vi "PL Model.vi"(7 "PL Model Exit":refnum<notifier>, 8 "error in (no error)":errorcluster, 10 "Controller queue":refnum<queue>, 11 "Message Queue In":refnum<queue>) -> (0 "error out":errorcluster)   [LabVIEW 2015, in "PL Model.lvlib"]
uses:
  PL Model.lvlib
  support/Message Queue/Message Cluster.ctl
  TypeDefs/UI/Line simulation.ctl
  TypeDefs/PL Model Data.ctl
  TypeDefs/PL Settings.ctl
  TypeDefs/PL UI Refs.ctl
  API/Get Model Status Control.ctl
  SubVIs/Global Data.vi
  support/Message Queue/Enqueue Message (Single).vi
  <vilib>/Utility/error.llb/Error Cluster From Error Code.vi
  <vilib>/ErrorRing/Error Ring.xnode
  support/Message Queue/PLC Message Queue.lvlib
  support/Message Queue/Message Queue.lvlib
panel:
  out "PL Model counter":i32
  out "Barrel Number":i32
  out "BARREL FILLED":bool
  out "SPILL ALARM":bool
  out "OUTPUT":bool
  out "DOSING":bool
  out "INPUT":bool
  out "Flow [l/s]":dbl(knob) scale=0.0..30.0
  out "Fluid Level [l]":dbl(slide) scale=0.0..100.0
  out "Production line":T1 max=100.0 scale=0.0..20.0
  out "Pump":bool
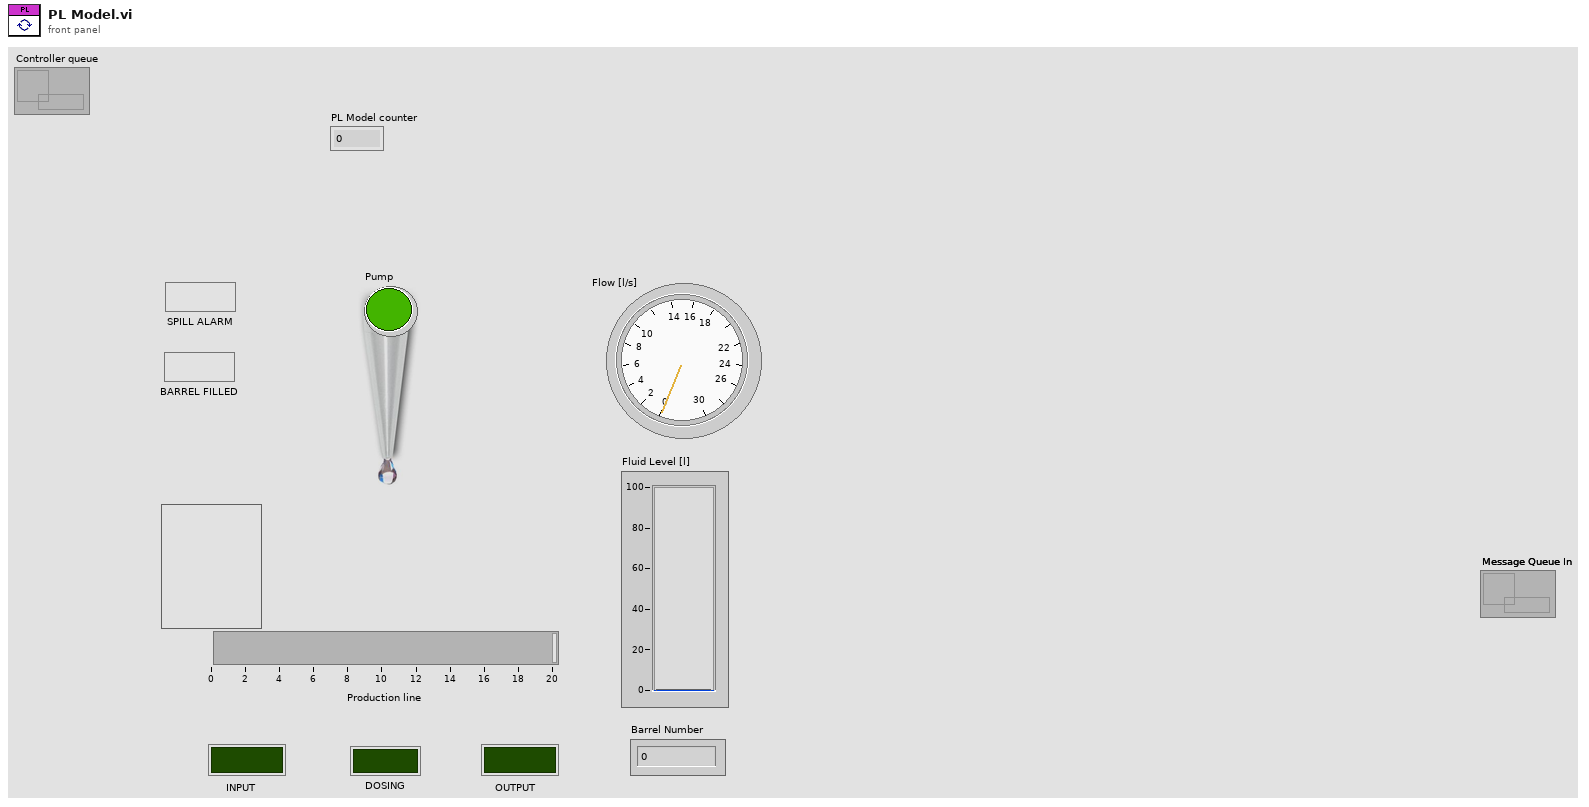
[diagram p1: front panel]
types:
  T1 = typedef "PL Model.lvlib/Line simulation.ctl" = dbl
  T2 = typedef "PL Model.lvlib/PL Model Data.ctl" = cluster{"Position":dbl, "Settings":T3, "Pump State":bool, "Fluid Flow":dbl, "Inpute Zone":bool, "Dosing Zone":bool, "Output Zone":bool, "UI Refs":T4, "Fluid Level":dbl, "Barrel Number":i32, "Spill Alarm":bool, "Level Alarm":bool, "millisecond timer value":u32}
  T3 = typedef "PL Model.lvlib/PL Settings.ctl" = cluster{"Length [m]":dbl, "Dose Zone Start":dbl, "Dose Zone  End":dbl, "Barrel Volume [l]":dbl, "Dosing level [l]":dbl}
  T4 = typedef "PL Model.lvlib/PL UI Refs.ctl" = cluster{"DOSING":refnum<vi>, "INPUT":refnum<vi>, "OUTPUT":refnum<vi>, "Pump":refnum<vi>, "Fluid Level [l]":refnum<vi>, "Flow [l/s]":refnum<vi>, "Production line":refnum<vi>, "SPILL":refnum<vi>, "LOW LEVEL":refnum<vi>, "Barrel Number":refnum<vi>}
  T5 = typedef "PL Model.lvlib/Get Model Status Control.ctl" = cluster{"Position":dbl, "Pump State":bool, "Fluid Flow":dbl, "Fluid Level":dbl, "Barrel Number":i32, "Spill Alarm":bool, "Level Alarm":bool}
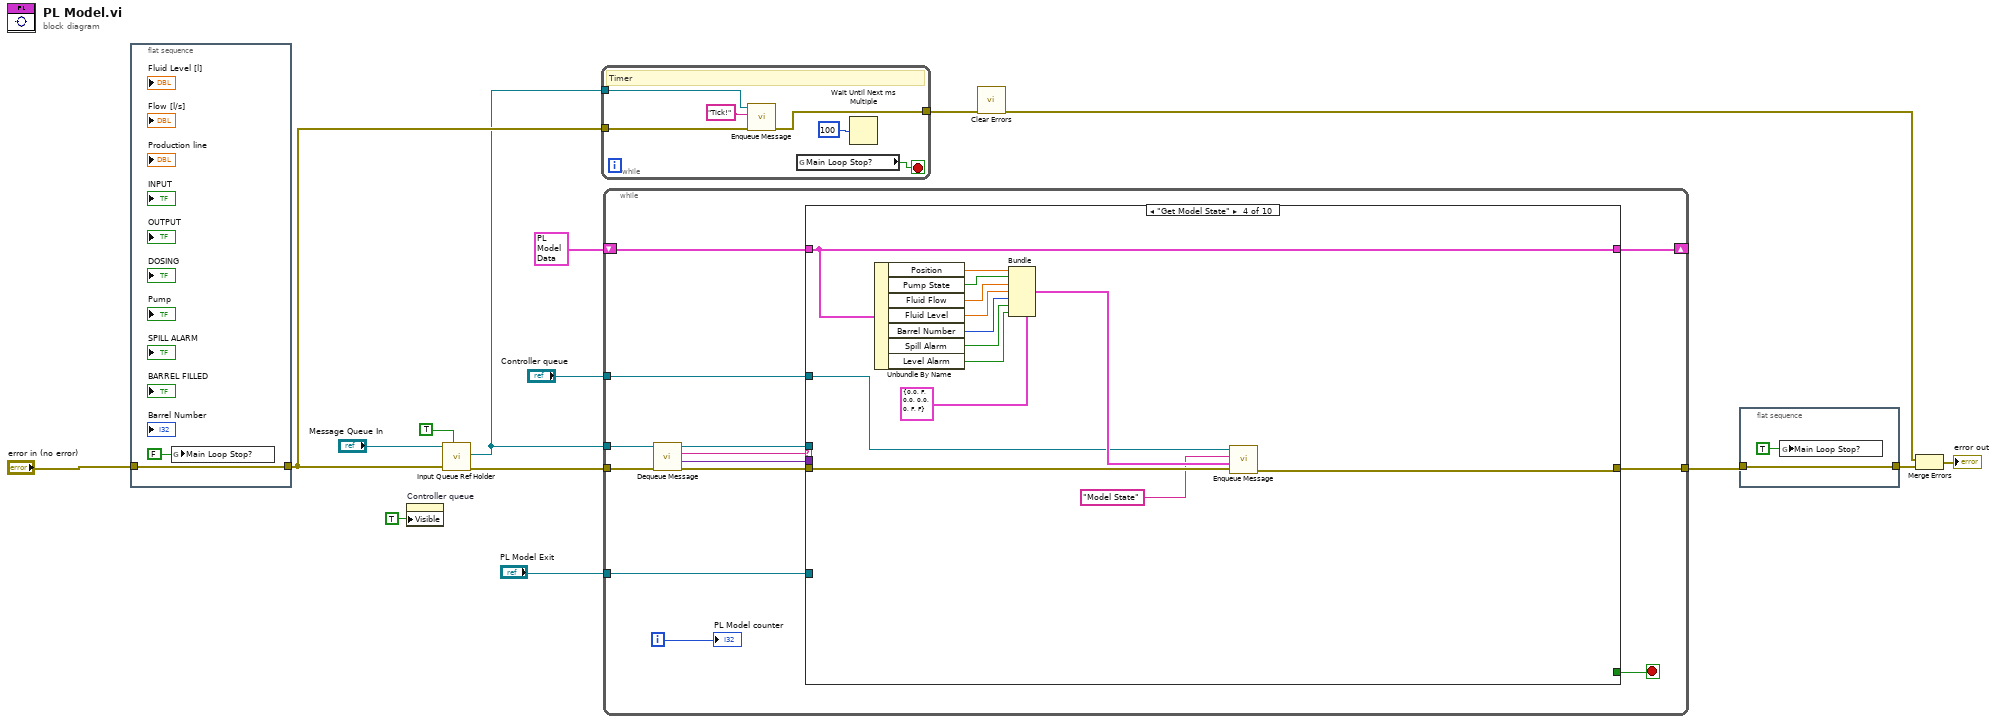
[diagram p0: block diagram]
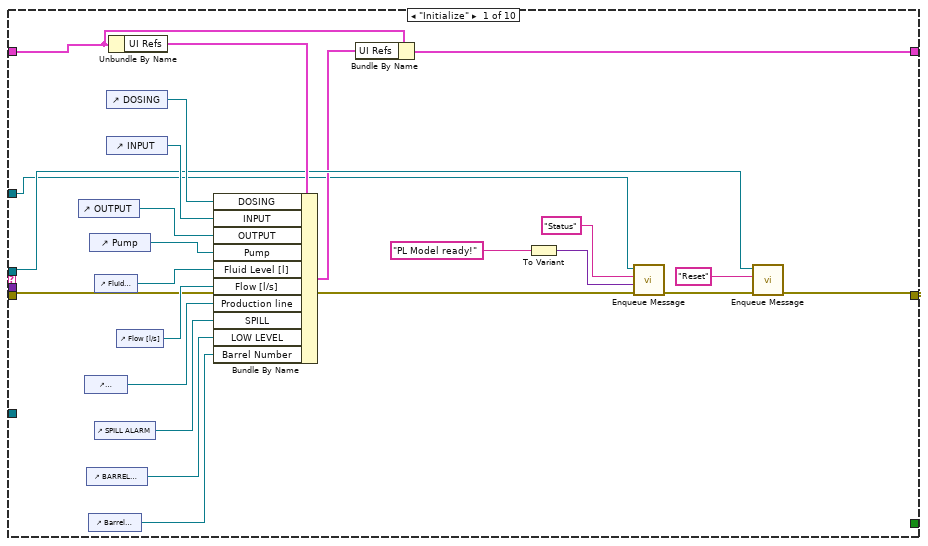
[diagram p2: hidden frame]
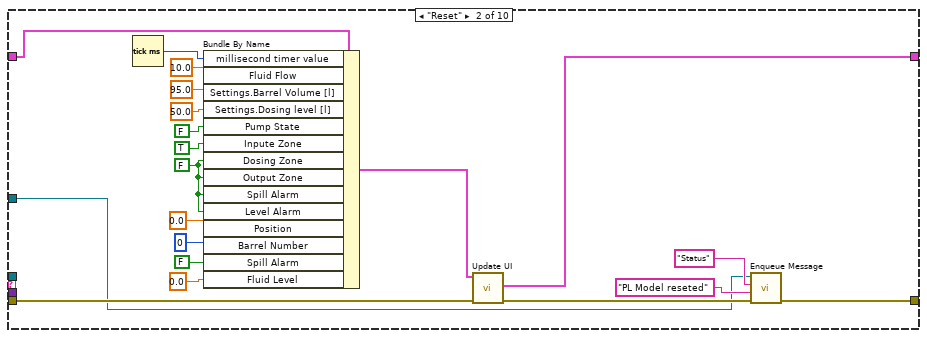
[diagram p3: hidden frame]
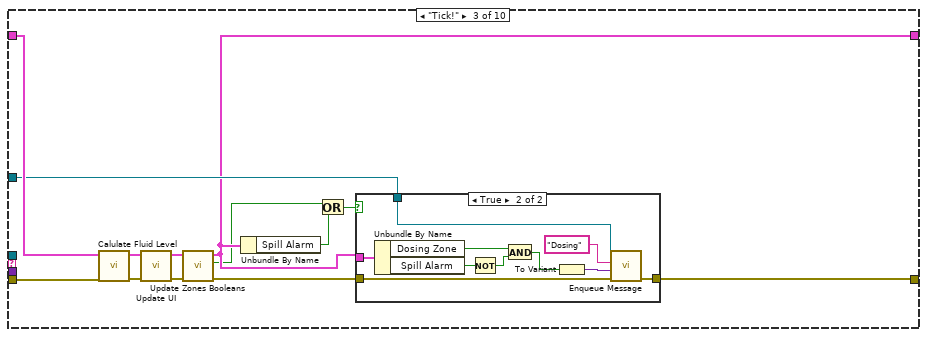
[diagram p4: hidden frame]
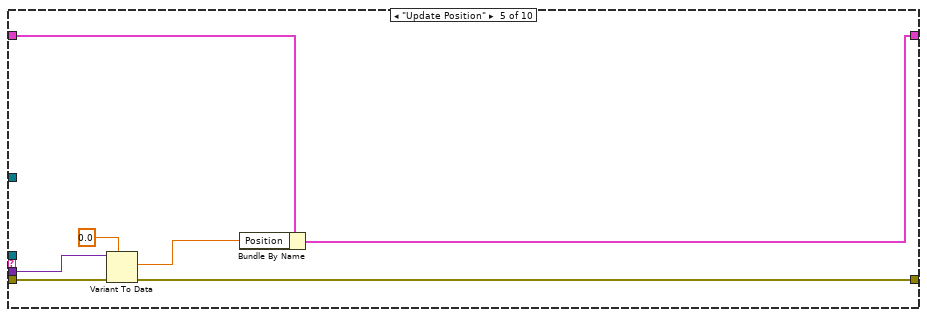
[diagram p6: hidden frame]
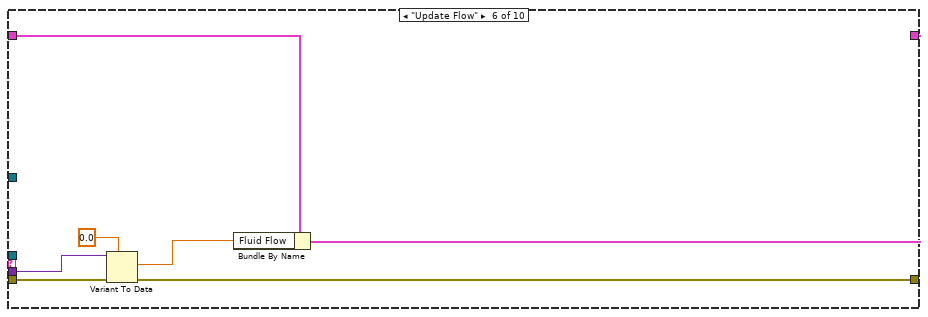
[diagram p7: hidden frame]
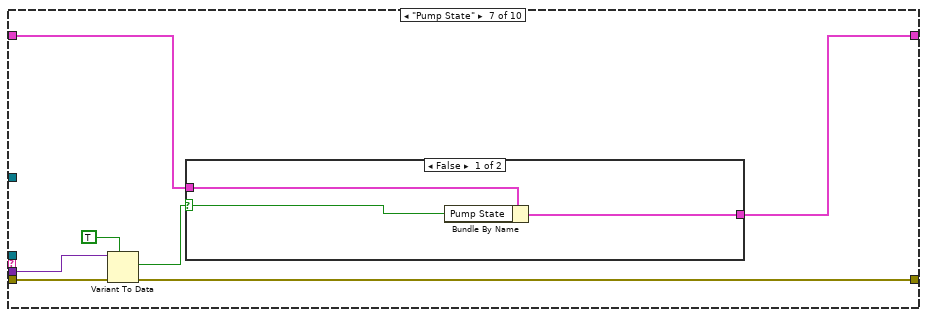
[diagram p8: hidden frame]
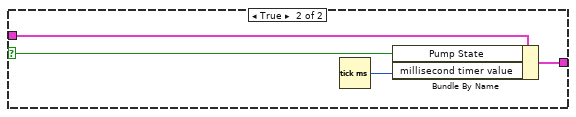
[diagram p9: hidden frame]
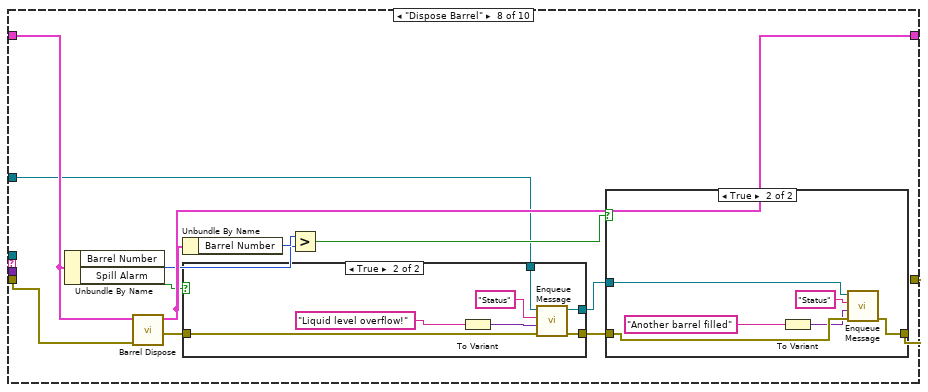
[diagram p10: hidden frame]
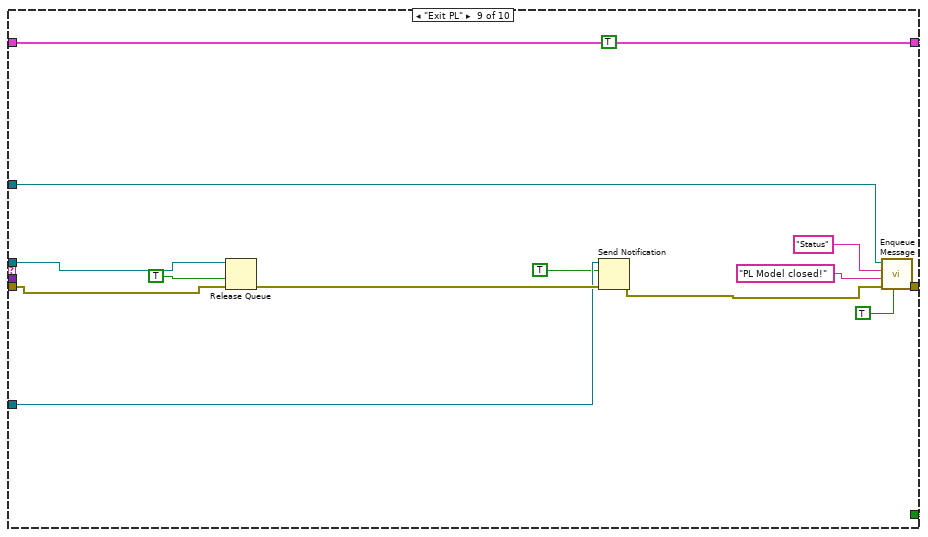
[diagram p13: hidden frame]
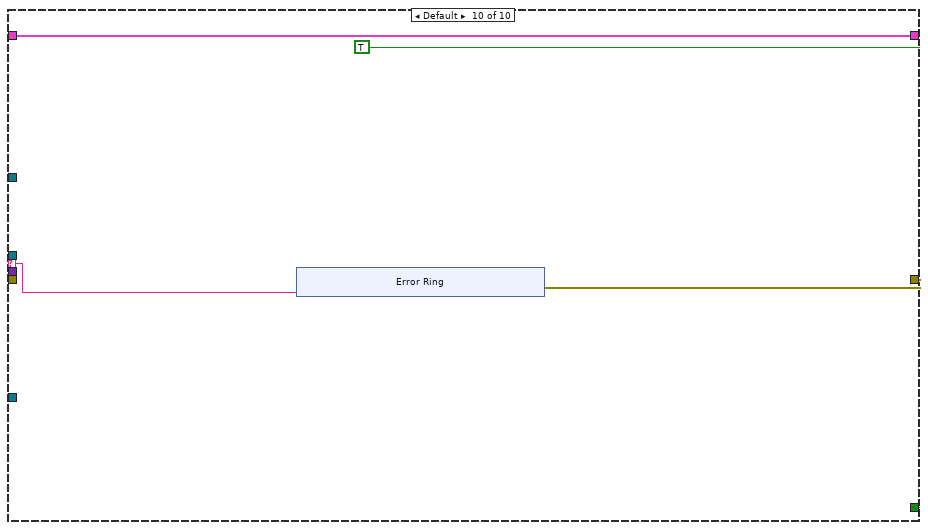
[diagram p14: hidden frame]
diagram:
  n1 = flat-sequence {
    tunnel: "error in (no error)" -> [w16]
    tunnel: [w16] -> w10
    frame #0 {
      n2 = global write "Global Data.vi" "Main Loop Stop?"(FALSE ("Main Loop Stop?")) -> ()
    }
  }
  n3 = property on="Controller queue" class="TypRef (strict)"("Visible"=TRUE) -> ()  [unwired: 2 in, 2 out]
  n4 = call "Input Queue Ref Holder.vi"("Hold"=TRUE, "error in (no error)"=w10, "Message Queue In"="Message Queue In") -> ("error out"=w9:errorcluster, "Input Message Queue"=w6:refnum<queue>)  [unwired: 7 in]
  n5 = while {
    tunnel: w6 -> [w21]
    tunnel: [w20] -> w3
    tunnel: w10 -> [w18]
    stop <- w22 stop-if-true
    # "Timer"
    n6 = call-poly "Enqueue Message.vi"("error in (no error)"=w18, "Message"="Tick!", "Message Queue"=w21) -> ("error out"=w20:errorcluster)  [unwired: 7 in, 1 out]
    n7 = global read "Global Data.vi" "Main Loop Stop?"() -> (w22:bool)
    n8 = Wait Until Next ms Multiple(millisecond multiple=u32 100) -> ()  [unwired: 1 out]
  }
  n9 = while {
    tunnel: w6 -> [w36]
    shift-right: [w28] -> _
    shift-left: T2 {"Position"=0.0, "Settings"={"Length [m]"=20.0, "Dose Zone Start"=8.0, "Dose Zone  End"=12.0, "Barrel Volume [l]"=100.0, "Dosing level [l]"=90.0}, "Pump State"=FALSE, "Fluid Flow"=0.0, "Inpute Zone"=FALSE, "Dosing Zone"=FALSE, "Output Zone"=FALSE, "UI Refs"={"DOSING"=refnum, "INPUT"=refnum, "OUTPUT"=refnum, "Pump"=refnum, "Fluid Level [l]"=refnum, "Flow [l/s]"=refnum, "Production line"=refnum, "SPILL"=refnum, "LOW LEVEL"=refnum, "Barrel Number"=refnum}, "Fluid Level"=0.0, "Barrel Number"=0, "Spill Alarm"=FALSE, "Level Alarm"=FALSE, "millisecond timer value"=0} ("PL Model Data") -> [w29]
    tunnel: [w34] -> w13
    tunnel: w9 -> [w33]
    tunnel: "PL Model Exit" -> [w26]
    tunnel: "Controller queue" -> [w25]
    i -> [w24]
    stop <- w27 stop-if-true
    n10 = call "Dequeue Message.vi"("error in (no error)"=w33, "Message Queue"=w36) -> ("error out"=w35:errorcluster, "Message Data"=w31:variant, "Message"=w32:string, "dup Message Queue"=w30:refnum<queue>)  [unwired: 6 in]
    n11 = case shown="\"Get Model State\"" w32 {
      selector: w32 -> [_ _ _ _ _ _ _ _ _ w191]
      tunnel: w35 -> [w37 w67 w92 w109 w124 w131 w138 w157 w185 _]
      tunnel: [w42 w68 w85 w108 w118 w125 w133 w156 w177 w190] -> w34
      tunnel: w31 -> [_ _ _ _ w123 w130 w137 _ _ _]
      tunnel: w30 -> [w44 _ _ _ _ _ _ _ w184 _]
      tunnel: w29 -> [w40 w79 w91 w107 w122 w129 w136 w155 w187 w188]
      tunnel: [w39 w65 w84 w107 w121 w128 w135 w154 w187 w188] -> w28
      tunnel: [_ _ _ _ _ _ _ _ TRUE TRUE] -> w27
      tunnel: w26 -> [_ _ _ _ _ _ _ _ w182 _]
      tunnel: w25 -> [w38 w60 w87 w105 _ _ _ w146 w174 _]
      frame "Initialize" {
        n12 = control-ref of="OUTPUT"() -> (w55:refnum<vi>)
        n13 = control-ref of="Production line"() -> (w59:refnum<vi>)
        n14 = control-ref of="BARREL FILLED"() -> (w51:refnum<vi>)
        n15 = control-ref of="Barrel Number"() -> (w49:refnum<vi>)
        n16 = control-ref of="Pump"() -> (w56:refnum<vi>)
        n17 = control-ref of="Fluid Level [l]"() -> (w57:refnum<vi>)
        n18 = control-ref of="SPILL ALARM"() -> (w50:refnum<vi>)
        n19 = control-ref of="DOSING"() -> (w53:refnum<vi>)
        n20 = control-ref of="INPUT"() -> (w54:refnum<vi>)
        n21 = Unbundle By Name(w40) -> ("UI Refs"=w52:T4)
        n22 = control-ref of="Flow [l/s]"() -> (w58:refnum<vi>)
        n23 = Bundle By Name(cluster=w52, "DOSING"=w53, "INPUT"=w54, "OUTPUT"=w55, "Pump"=w56, "Fluid Level [l]"=w57, "Flow [l/s]"=w58, "Production line"=w59, "SPILL"=w50, "LOW LEVEL"=w51, "Barrel Number"=w49) -> (w41:T4)
        n24 = Bundle By Name(cluster=w40, "UI Refs"=w41) -> (w39:T2)
        n25 = To Variant(anything="PL Model ready!" ("Message")) -> (Variant=w46:variant)
        n26 = call-poly "Enqueue Message.vi"("error in (no error)"=w37, "Message Data"=w46, "Message"="Status", "Message Queue"=w38) -> ("error out"=w45:errorcluster)  [unwired: 6 in, 1 out]
        n27 = call-poly "Enqueue Message.vi"("error in (no error)"=w45, "Message"="Reset", "Message Queue"=w44) -> ("error out"=w42:errorcluster)  [unwired: 7 in, 1 out]
      }
      frame "Reset" {
        w71 = FALSE ("Inpute Zone")
        n28 = Tick Count (ms)() -> (millisecond timer value=w76:u32)
        n29 = Bundle By Name(cluster=w79, "millisecond timer value"=w76, "Fluid Flow"=10.0, "Settings.Barrel Volume [l]"=95.0, "Settings.Dosing level [l]"=50.0, "Pump State"=FALSE, "Inpute Zone"=TRUE, "Dosing Zone"=w71, "Output Zone"=w71, "Spill Alarm"=w71, "Level Alarm"=w71, "Position"=0.0, "Barrel Number"=0, "Spill Alarm"=FALSE, "Fluid Level"=0.0) -> (w69:T2)
        n30 = call "Update UI.vi"("error in (no error)"=w67, "PL Model Data"=w69) -> ("error out"=w66:errorcluster, "PL Model Data"=w65:T2)  [unwired: 8 in]
        n31 = call-poly "Enqueue Message.vi"("error in (no error)"=w66, "Message Data"="PL Model reseted" ("Message"), "Message"="Status", "Message Queue"=w60) -> ("error out"=w68:errorcluster)  [unwired: 6 in, 1 out]
      }
      frame "Tick!" {
        n32 = call "Calulate Fluid Level.vi"("error in (no error)"=w92, "PL Model Data"=w91) -> ("error out"=w90:errorcluster, "PL Model Data Out"=w80:T2)  [unwired: 8 in]
        n33 = call "Update UI.vi"("error in (no error)"=w90, "PL Model Data"=w80) -> ("error out"=w89:errorcluster, "PL Model Data"=w88:T2)  [unwired: 8 in]
        n34 = call "Update Zones Booleans.vi"("error in (no error)"=w89, "PL Model Data"=w88) -> ("error out"=w86:errorcluster, "Zone change?"=w83:bool, "PL Model Data 2"=w84:T2)  [unwired: 7 in]
        n35 = Unbundle By Name(w84) -> ("Spill Alarm"=w81:bool)
        n36 = Or(x=w83, y=w81) -> (x .or. y?=w82:bool)
        n37 = case shown="True" w82 {
          tunnel: w84 -> [_ w103]
          tunnel: w87 -> [_ w102]
          tunnel: w86 -> [w93 w101]
          tunnel: [w93 w94] -> w85
          frame False {
          }
          frame True {
            n38 = Unbundle By Name(w103) -> ("Dosing Zone"=w96:bool, "Spill Alarm"=w98:bool)
            n39 = Not(x=w98) -> (.not. x?=w97:bool)
            n40 = And(x=w96, y=w97) -> (x .and. y?=w95:bool)
            n41 = To Variant(anything=w95) -> (Variant=w100:variant)
            n42 = call-poly "Enqueue Message.vi"("error in (no error)"=w101, "Message Data"=w100, "Message"="Dosing", "Message Queue"=w102) -> ("error out"=w94:errorcluster)  [unwired: 6 in, 1 out]
          }
        }
      }
      frame "Get Model State" {
        n43 = Unbundle By Name(w107) -> ("Position"=w117:dbl, "Pump State"=w116:bool, "Fluid Flow"=w115:dbl, "Fluid Level"=w114:dbl, "Barrel Number"=w113:i32, "Spill Alarm"=w112:bool, "Level Alarm"=w111:bool)
        n44 = Bundle(cluster=T5 {"Position"=0.0, "Pump State"=FALSE, "Fluid Flow"=0.0, "Fluid Level"=0.0, "Barrel Number"=0, "Spill Alarm"=FALSE, "Level Alarm"=FALSE} ("output cluster"), "Position"=w117, "Pump State"=w116, "Fluid Flow"=w115, "Fluid Level"=w114, "Barrel Number"=w113, "Spill Alarm"=w112, "Level Alarm"=w111) -> (w106:T5)
        n45 = call-poly "Enqueue Message.vi"("error in (no error)"=w109, "Message Data"=w106, "Message"="Model State", "Message Queue"=w105) -> ("error out"=w108:errorcluster)  [unwired: 6 in, 1 out]
      }
      frame "Update Position" {
        n46 = Variant To Data(error in=w124, type=0.0, Variant=w123) -> (data=w119:dbl, error out=w118:errorcluster)
        n47 = Bundle By Name(cluster=w122, "Position"=w119) -> (w121:T2)
      }
      frame "Update Flow" {
        n48 = Variant To Data(error in=w131, type=0.0, Variant=w130) -> (data=w126:dbl, error out=w125:errorcluster)
        n49 = Bundle By Name(cluster=w129, "Fluid Flow"=w126) -> (w128:T2)
      }
      frame "Pump State" {
        n50 = Variant To Data(error in=w138, type=TRUE, Variant=w137) -> (data=w132:bool, error out=w133:errorcluster)
        n51 = case shown="False" w132 {
          selector: w132 -> [w139 w142]
          tunnel: w136 -> [w141 w145]
          tunnel: [w140 w144] -> w135
          frame False {
            n52 = Bundle By Name(cluster=w141, "Pump State"=w139) -> (w140:T2)
          }
          frame True {
            n53 = Tick Count (ms)() -> (millisecond timer value=w143:u32)
            n54 = Bundle By Name(cluster=w145, "Pump State"=w142, "millisecond timer value"=w143) -> (w144:T2)
          }
        }
      }
      frame "Dispose Barrel" {
        n55 = Unbundle By Name(w155) -> ("Barrel Number"=w152:i32, "Spill Alarm"=w147:bool)
        n56 = call "Barrel Dispose.vi"("error in (no error)"=w157, "PL Model Data in"=w155) -> ("error out"=w149:errorcluster, "PL Model Data out"=w154:T2)  [unwired: 8 in]
        n57 = Unbundle By Name(w154) -> ("Barrel Number"=w153:i32)
        n58 = case shown="True" w147 {
          tunnel: w149 -> [w159 w164]
          tunnel: [w159 w163] -> w148
          tunnel: [w158 w162] -> w150
          tunnel: w146 -> [w158 w160]
          frame False {
          }
          frame True {
            n59 = To Variant(anything="Liquid level overflow!" ("Message")) -> (Variant=w161:variant)
            n60 = call-poly "Enqueue Message.vi"("error in (no error)"=w164, "Message Data"=w161, "Message"="Status", "Message Queue"=w160) -> ("error out"=w163:errorcluster, "dup Message Queue"=w162:refnum<queue>)  [unwired: 6 in]
          }
        }
        n61 = Greater?(x=w153, y=w152) -> (0:w151:bool)
        n62 = case shown="True" w151 {
          tunnel: w150 -> [_ w171]
          tunnel: w148 -> [w167 w170]
          tunnel: [w167 w169] -> w156
          frame False {
          }
          frame True {
            n63 = To Variant(anything="Another barrel filled" ("Message")) -> (Variant=w168:variant)
            n64 = call-poly "Enqueue Message.vi"("error in (no error)"=w170, "Message Data"=w168, "Message"="Status", "Message Queue"=w171) -> ("error out"=w169:errorcluster)  [unwired: 6 in, 1 out]
          }
        }
      }
      frame "Exit PL" {
        n65 = Release Queue(queue=w184, force destroy? (F)=TRUE, error in (no error)=w185) -> (error out=w183:errorcluster)  [unwired: 2 out]
        n66 = Send Notification(notification=TRUE, notifier=w182, error in (no error)=w183) -> (error out=w178:errorcluster)  [unwired: 1 out]
        n67 = call-poly "Enqueue Message.vi"("Priority Message? (F)"=TRUE, "error in (no error)"=w178, "Message Data"="PL Model closed!" ("Message"), "Message"="Status", "Message Queue"=w174) -> ("error out"=w177:errorcluster)  [unwired: 5 in, 1 out]
      }
      frame Default {
        n68 = xnode "Error Ring"("parameter 0"=w191) -> ("error out"=w190:errorcluster)
      }
    }
    "PL Model counter" <- w24
  }
  n69 = call <vilib>:"Clear Errors.vi"("error in (no error)"=w3) -> ("error out"=w2:errorcluster)  [unwired: 5 in, 1 out]
  n70 = flat-sequence {
    tunnel: w13 -> [w199]
    tunnel: [w199] -> w12
    frame #0 {
      n71 = global write "Global Data.vi" "Main Loop Stop?"(TRUE ("Main Loop Stop?")) -> ()
    }
  }
  n72 = Merge Errors(w2, w12) -> (→"error out":errorcluster)
